vi "sendCmdAndLog.vi"(8 "error in (no error)":errorcluster, 9 "working directory":path, 10 "command":string) -> (0 "error out":errorcluster, 1 "Log":string, 2 "standard output":string)   [LabVIEW 2013, in "hgHandler.lvclass"]
uses:
  hgHandler.lvclass
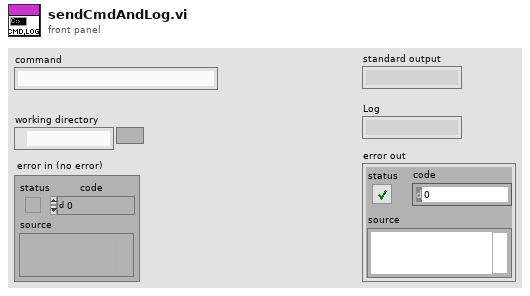
[diagram p1: front panel]
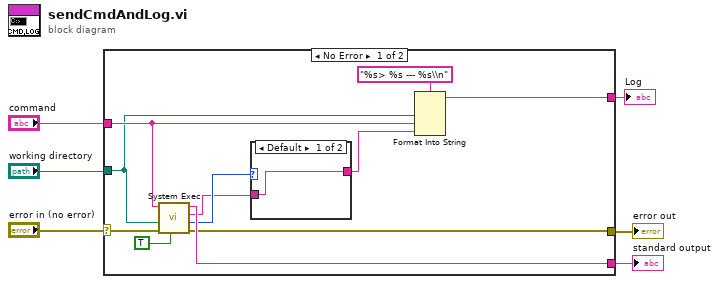
[diagram p0: block diagram]
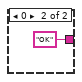
[diagram p2: hidden frame]
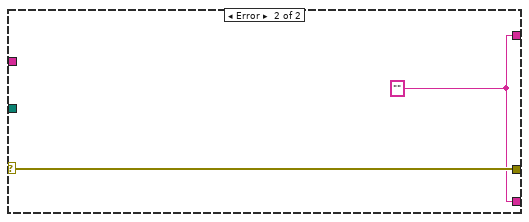
[diagram p3: hidden frame]
diagram:
  n1 = case shown="No Error" "error in (no error)" {
    selector: "error in (no error)" -> [w16 w21]
    tunnel: [w8 w21] -> w6
    tunnel: "command" -> [w11 _]
    tunnel: [w15 w20] -> w3
    tunnel: "working directory" -> [w9 _]
    tunnel: [w7 w20] -> w1
    frame No Error {
      n2 = call <vilib>:"System Exec.vi"("run minimized? (F)"=TRUE, "error in (no error)"=w16, "working directory"=w9, "command line"=w11) -> ("error out"=w8:errorcluster, "return code"=w14:i32, "standard error"=w13:string, "standard output"=w15:string)  [unwired: 4 in]
      n3 = case shown="Default" w14 {
        tunnel: w13 -> [w18 _]
        tunnel: [w18 "OK" ("standard error")] -> w10
        frame Default {
        }
        frame 0 {
        }
      }
      n4 = Format Into String(format string="%s> %s --- %s\\n", w9, w11, w10) -> (resulting string=w7:string)  [unwired: 2 in, 1 out]
    }
    frame Error {
      w20 = "" ("standard output")
    }
  }
  "error out" <- w6
  "standard output" <- w3
  "Log" <- w1
